vi "HaveLegalPosition.vi"(5 "ChessBoard":T1, 9 "StoneColor":u16) -> (8 "HaveLegalPlace?":bool)   [LabVIEW 2009]
doc: "To judge if there is a Legal place.\nLegal: Empty and can move stone on."
uses:
  Controls/Chess.ctl
  Controls/ItemIndex.ctl
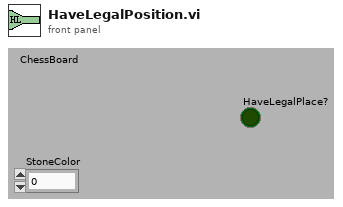
[diagram p1: front panel]
types:
  T1 = typedef "Chess.ctl" = u16[][]
  T2 = typedef "ItemIndex.ctl" = cluster{"Row":i32, "Col":i32}
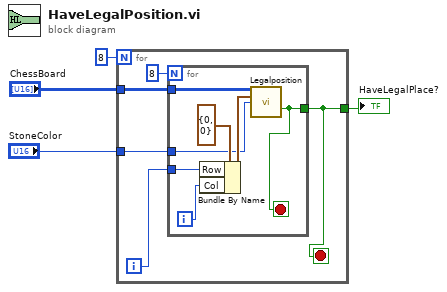
[diagram p0: block diagram]
diagram:
  n1 = for {
    N: 8 -> [_]
    tunnel: "ChessBoard" -> [w7]
    tunnel: "StoneColor" -> [w6]
    tunnel: [w5] -> w4
    i -> [w9]
    stop <- w5 stop-if-true
    n2 = for {
      N: 8 -> [_]
      tunnel: w9 -> [w14]
      tunnel: w7 -> [w16]
      tunnel: w6 -> [w11]
      tunnel: [w10] -> w5
      i -> [w13]
      stop <- w10 stop-if-true
      n3 = Bundle By Name(cluster=T2 {"Row"=0, "Col"=0} ("ItemIndex"), "Row"=w14, "Col"=w13) -> (w15:T2)
      n4 = call "Legalposition.vi"("Chessboard"=w16, "ItemIndex"=w15, "StoneColor"=w11) -> ("Legal?"=w10:bool)  [unwired: 8 in, 4 out]
    }
  }
  "HaveLegalPlace?" <- w4
